vi "Shutdown Components.vi"(8 "error in (no error)":errorcluster, 11 "Transceiver Thread in":refnum<class "Transceiver Thread.lvclass">) -> (0 "error out":errorcluster, 3 "Transceiver Thread out":refnum<class "Transceiver Thread.lvclass">)   [LabVIEW 2020, in "DSF Core.lvlib" / "Transceiver Thread.lvclass"]
uses:
  Transceiver Thread.lvclass
  Transceiver Thread.lvclass/Transceiver Thread.ctl
  Transceiver/Transceiver.lvclass
  Buffer Converter/Buffer Converter.lvclass
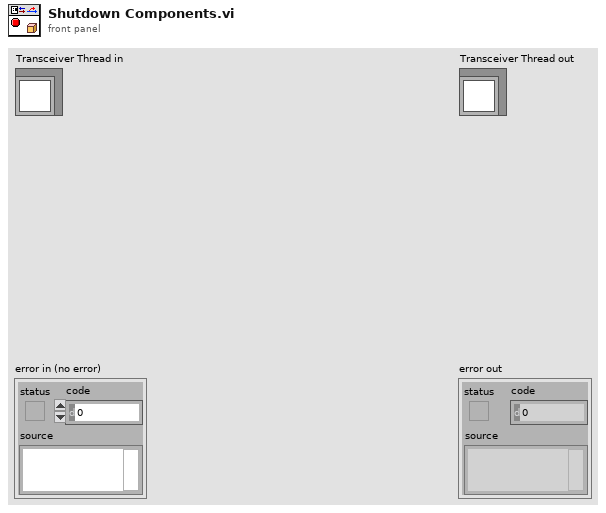
[diagram p1: front panel]
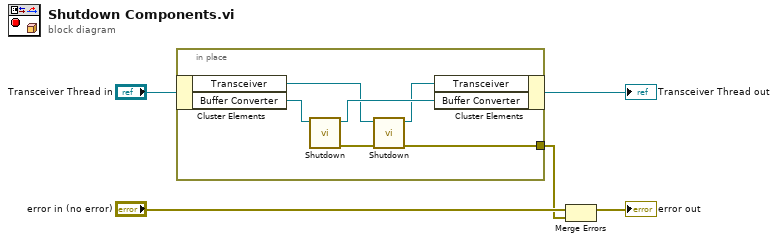
[diagram p0: block diagram]
diagram:
  n1 = in-place {
    in-place-border: [w6] -> w2
    n2 = in-place-cluster #1("Transceiver Thread in") -> ("Transceiver"=w8:refnum<class "Transceiver.lvclass">, "Buffer Converter"=w11:refnum<class "Buffer Converter.lvclass">)
    n3 = call-dynamic "Shutdown.vi"("Buffer Converter in"=w11) -> ("error out"=w10:errorcluster, "Buffer Converter out"=w9:refnum<class "Buffer Converter.lvclass">)  [unwired: 9 in]
    n4 = call-dynamic "Shutdown.vi"("error in (no error)"=w10, "Transceiver in"=w8) -> ("error out"=w6:errorcluster, "Transceiver out"=w7:refnum<class "Transceiver.lvclass">)  [unwired: 8 in]
    n5 = in-place-cluster #1("Transceiver"=w7, "Buffer Converter"=w9) -> (→"Transceiver Thread out":refnum<class "Transceiver Thread.lvclass">)
  }
  n6 = Merge Errors("error in (no error)", w2) -> (→"error out":errorcluster)
